vi "Class_Tree Tag_Decode.vi"(11 "Tag In":string) -> (3 "TagData":T1)   [LabVIEW 2023]
doc: "Decode from tree tag the unique ID string for a method or property, and return the short and long names. The long name is the colon-dlimited name as it appears in the property node. The short name is the value afte the colon, eg:\n\nLong = Bounds:Legnth\nShort = Legnth\nParent= Bounds"
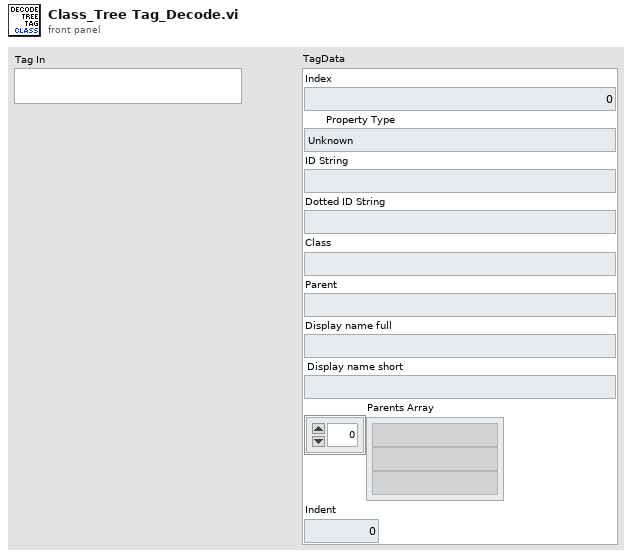
[diagram p1: front panel]
types:
  T1 = cluster{"Index":u16, "Property Type":enum16{"Unknown", "Base", "Scripting", "Private", "Deprecated", "None", "Divider"}, "ID String":string, "Dotted ID String":string, "Class":string, "Parent":string, "Display name full":string, "Display name short":string, "Parents Array":string[], "Indent":u16}
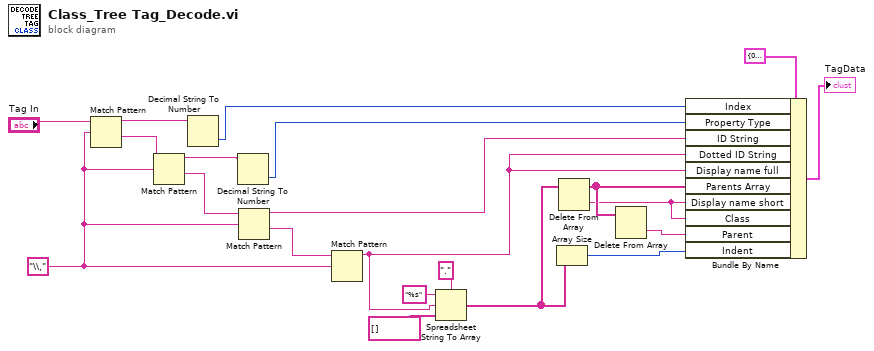
[diagram p0: block diagram]
diagram:
  w16 = "\\," ("search string")
  n1 = Match Pattern(string="Tag In", regular expression=w16) -> (before substring=w20:string, after substring=w19:string)  [unwired: 1 in, 2 out]
  n2 = Match Pattern(string=w19, regular expression=w16) -> (before substring=w17:string, after substring=w18:string)  [unwired: 1 in, 2 out]
  n3 = Decimal String To Number(string=w20) -> (number=w14:i32)  [unwired: 2 in, 1 out]
  n4 = Decimal String To Number(string=w17) -> (number=w13:i32)  [unwired: 2 in, 1 out]
  n5 = Match Pattern(string=w18, regular expression=w16) -> (before substring=w12:string, after substring=w15:string)  [unwired: 1 in, 2 out]
  n6 = Match Pattern(string=w15, regular expression=w16) -> (before substring=w3:string)  [unwired: 1 in, 3 out]
  n7 = Spreadsheet String To Array(delimiter (Tab)=".", format string="%s", spreadsheet string=w3, array type (2D Dbl)=string[] [] ("format string")) -> (array=w5:string[])
  n8 = Array Size(array=w5) -> (size(s)=w6:i32)
  n9 = Delete From Array(array=w5) -> (deleted portion=w1:string, array with subset deleted=w4:string[])  [unwired: 2 in]
  n10 = Delete From Array(array=w4) -> (deleted portion=w2:string)  [unwired: 2 in, 1 out]
  n11 = Bundle By Name(cluster=T1 {"Index"=0, "Property Type"=enum."Unknown", "ID String"="", "Dotted ID String"="", "Class"="", "Parent"="", "Display name full"="", "Display name short"="", "Parents Array"=[], "Indent"=0} ("TagData"), "Index"=w14, "Property Type"=w13, "ID String"=w12, "Dotted ID String"=w3, "Display name full"=w3, "Parents Array"=w4, "Display name short"=w1, "Class"=w1, "Parent"=w2, "Indent"=w6) -> (→"TagData":T1)
